vi "GetWaypoints.vi"() -> (2 "Waypoint Index":dbl, 3 "Waypoints":cluster{"Longitude":dbl, "Latitude":dbl}[](array[cluster]))   [LabVIEW 2011]
uses:
  <vilib>/Utility/file.llb/Read From Spreadsheet File (DBL).vi
panel:
  in  "file path (dialog if empty)":path=path "C:/Users/Robot/Desktop/Robot VIs (organized)"
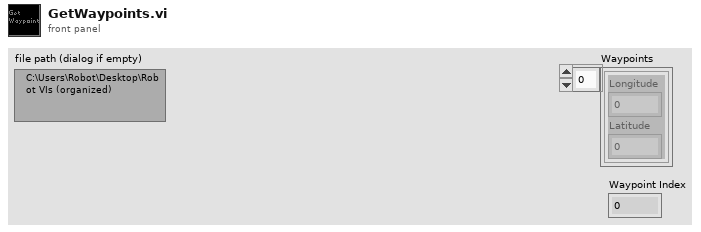
[diagram p1: front panel]
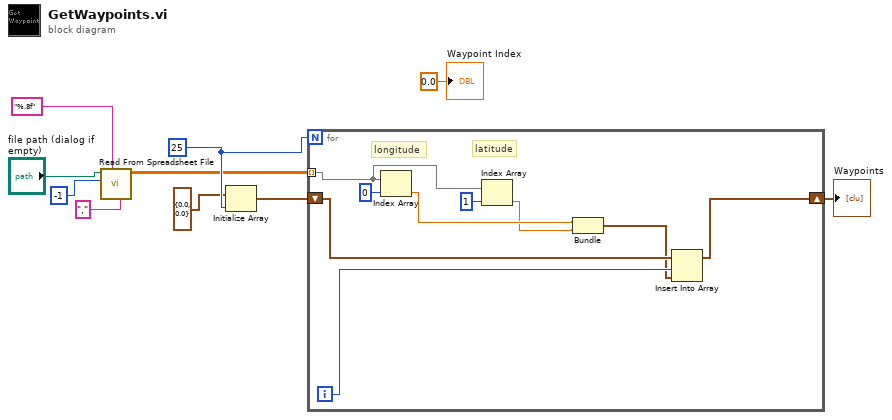
[diagram p0: block diagram]
diagram:
  w10 = 25 ("dimension size")
  n1 = call-poly <vilib>:"Read From Spreadsheet File.vi"("delimiter (\\t)"="," ("delimiter (\\t)"), "format (%.3f)"="%.8f", "number of rows (all:-1)"=-1, "file path (dialog if empty)"="file path (dialog if empty)") -> ("all rows"=w7:dbl[][])  [unwired: 3 in, 4 out]
  n2 = Initialize Array(cluster{"Longitude":dbl, "Latitude":dbl} {"Longitude"=0.0, "Latitude"=0.0} ("Robot Position"), w10) -> (w9:cluster{"Longitude":dbl, "Latitude":dbl}[])
  n3 = for {
    N: w10 -> [_]
    shift-right: [w11] -> w3
    shift-left: w9 -> [w16]
    tunnel: w7 -> [w17] mode=indexing
    i -> [w15]
    # "latitude"
    # "longitude"
    n4 = Index Array(array=w17, index=0) -> (element=w14:dbl)
    n5 = Index Array(array=w17, index=1) -> (element=w13:dbl)
    n6 = Bundle(w14, w13) -> (w12:cluster{dbl, dbl})  [unwired: 1 in]
    n7 = Insert Into Array(array=w16, index=w15, new element=w12) -> (w11:cluster{"Longitude":dbl, "Latitude":dbl}[])
  }
  "Waypoints" <- w3
  "Waypoint Index" <- 0.0 ("Waypoint Index")
